vi "To Waveform.vi"(8 "error in (no error)":errorcluster, 11 "Request Data in":refnum<class "Request Data.lvclass">) -> (0 "error out":errorcluster, 1 "Success?":bool, 3 "Waveform Array":waveform(dbl)[](array[waveform]))   [LabVIEW 2020, in "Publisher.lvlib" / "Request Data.lvclass"]
doc: "Interpret 'Data' as a Waveform Array. If impossible 'Success?' is set to FALSE"
uses:
  Request Data.lvclass
  Request Data.lvclass/Request Data.ctl
  PPL/HDH.Data.Generic.lvlibp/Data.lvclass
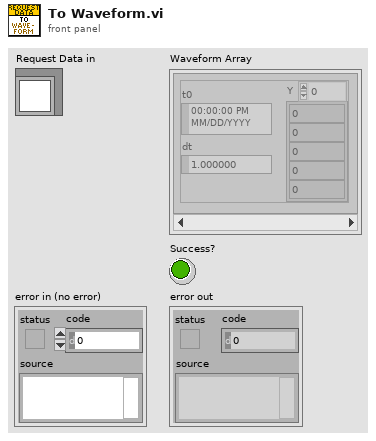
[diagram p1: front panel]
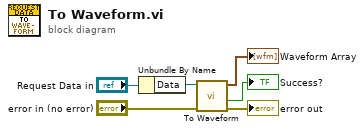
[diagram p0: block diagram]
diagram:
  n1 = Unbundle By Name("Request Data in") -> ("Data"=w5:refnum<class "Data.lvclass">)
  n2 = call-dynamic "To Waveform.vi"("error in (no error)"="error in (no error)", "Data in"=w5) -> ("error out"=→"error out":errorcluster, "Success?"=→"Success?":bool, "Waveform Array"=→"Waveform Array":waveform(dbl)[])  [unwired: 7 in]
